vi "Wait-for-action.vi"(8 "error in (no error)":errorcluster, 11 "Data ref. in":refnum<data-value>) -> (0 "error out":errorcluster, 2 "Next action":T1, 3 "Data ref.":refnum<data-value>)   [LabVIEW 2013, in "CameraVision.lvlib" / "CV-Main.lvclass"]
uses:
  CV-Main.lvclass
  Main-actions.ctl
  CV-Main.lvclass/CV-Main.ctl
  Read Action queue.vi
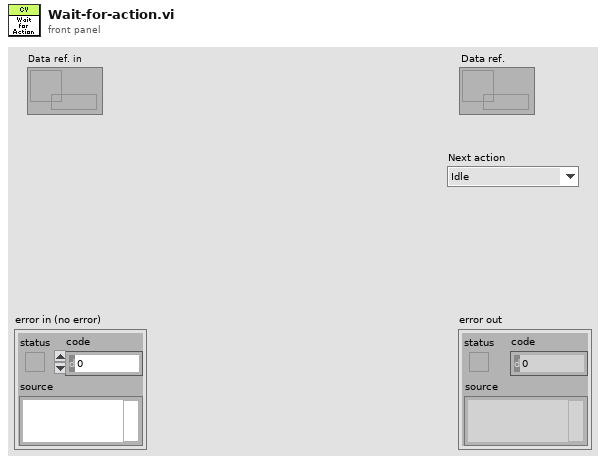
[diagram p1: front panel]
types:
  T1 = typedef "CameraVision.lvlib/CV-Main.lvclass/Main-actions.ctl" = enum16{"Idle", "Initialize", "Load defaults", "Update settings", "Check settings", "Save settings", "Save settings with dialog", "Load settings", "Load data", "Activate", "Start", "Wait for start signal", "Acquire & process", "Iterate", "Stop", "Refresh display", "Refresh status", "View camera settings", "View grabber settings", "Exit"}
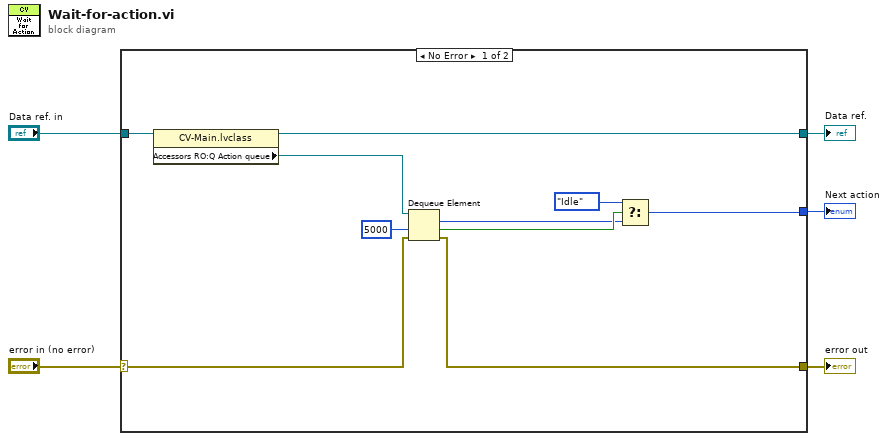
[diagram p0: block diagram]
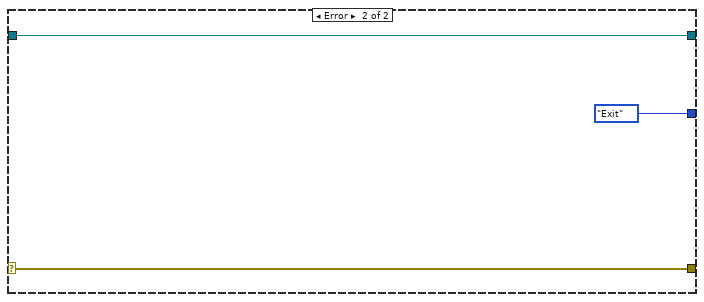
[diagram p2: hidden frame]
diagram:
  n1 = case shown="No Error" "error in (no error)" {
    selector: "error in (no error)" -> [w11 w18]
    tunnel: [w13 w18] -> w4
    tunnel: "Data ref. in" -> [w15 w17]
    tunnel: [w14 w17] -> w2
    tunnel: [w6 Main-actions."Exit" ("Main actions")] -> w1
    frame No Error {
      n2 = property class="CV-Main.lvclass"(reference=w15) -> (reference out=w14:refnum<data-value>, "Accessors RO:Q Action queue"=w10:refnum<queue>)  [unwired: 1 in, 1 out]
      n3 = Dequeue Element(queue=w10, timeout in ms (-1)=5000, error in (no error)=w11) -> (element=w8:T1, timed out?=w9:bool, error out=w13:errorcluster)  [unwired: 1 out]
      n4 = Select(t=Main-actions."Idle" ("Program status"), s=w9, f=w8) -> (s? t:f=w6:T1)
    }
    frame Error {
    }
  }
  "error out" <- w4
  "Data ref." <- w2
  "Next action" <- w1
